vi "GUI_HTT_save.vi"() -> ()   [LabVIEW 2013]
uses:
  shared programs/GUI_Template/GUI_master/tcp_new_data_event.ctl
  shared programs/GUI_Template/GUI_master/tcp new data cluster.ctl
  GUI_TestStand/Fire button.ctl
panel:
  in  "Position.Axis 3::5 2":dbl caption="Mode Out z" min=-200.0 max=200.0
  in  "Position.Axis 1::4":dbl caption="Blade" min=-20.0 max=20.0
  out "Temperature::11":dbl min=0.0 max=500.0 format="%#_3f"
  out "Temperature::10":dbl min=0.0 max=500.0 format="%#_3f"
  out "Energy.Channel 0::7":dbl min=0.0 max=20.0 format="%#_3e"
  in  "Amplitude.Ch 5::8":dbl caption="Trigger Amplitude" min=0.0 max=12.0
  in  "Position.Axis 3::5":dbl caption="Mode In z" min=-200.0 max=200.0
  in  "Position.Axis 1::5":dbl caption="Mode Out Wedge" min=-150.0 max=150.0
  out "Position.Axis3::2":dbl caption="Rotation G1" min=-180.0 max=180.0 format="%#_13g"
  out "Position.Axis2::2":dbl caption="Rotation G2" min=-180.0 max=180.0 format="%#_13g"
  in  "Position.Axis1::2":dbl caption="Translation" min=-60000.0 max=60000.0 format="%#_13g"
  in  "PicoL":bool caption="PicoL GUI"
  in  "PicoB":bool caption="PicoB GUI"
  in  "AnalogOutput.Channel 0::9":dbl caption="Pressure Ctrl (V)" min=0.0 max=10.0
  in  "Width.Ch 5::8":dbl caption="Opening time (s)" min=0.0 max=0.025 format="%#_6e"
  in  "Jet enable":bool caption="Jet Enable"
  in  "Jet trigger":bool caption="Jet Trigger"
  in  "Position.Axis 3::3":dbl caption="Jet z" min=0.0 max=25.0
  in  "Position.Axis 2::3":dbl caption="Jet y" min=0.0 max=25.0
  in  "Position.Axis 1::3":dbl caption="Jet X" min=0.0 max=25.0
  in  "Position.Axis 3::6":dbl caption="Probe delay" min=-76.0 max=76.0
  in  "GUIdevice 11":string="HTT-Temp-Amps"
  in  "GUIdevice 8":string="HTT-BNC"
  in  "GUIdevice 6":string="HTT-ESP04"
  in  "GUIdevice 5":string="HTT-ESP03"
  in  "Fire Button":T1=TRUE
  out "error IO 2":errorcluster
  out "fire::10":string
  out "tcp data event":T2
  in  "UDP error message":string
  in  "GUIdevice 7":string="HTT-Pulsar"
  in  "GUIdevice 2":string="HTT-Aerotech"
  in  "GUIdevice 10":string="HTT-Temp-Gaia"
  in  "GUIdevice 4":string="HTT-ESP02"
  in  "GUIdevice 1":string="U_1Wire_148"
  in  "GUIdevice 3":string="HTT-ESP01"
  in  "GUIdevice 9":string="HTT-HighPressureDAQ"
  in  "Delay.Ch 5::8":dbl caption="Jet timing (s)" min=0.0 max=10.0 format="%#_6e"
  in  "stop":bool
  # "Energy"
  # "CAP"
  # "HTT CONTROL CENTER"
  # "Drive"
  # "Gas Jet"
  # "Compressor"
  # "Mode Imager"
  # "Temp Gaia"
  # "Temp Amp"
  # "Energy"
  # "Prepulse Delay"
  # "Scatter (soon)"
  # "GUI Collection"
  # "Probe"
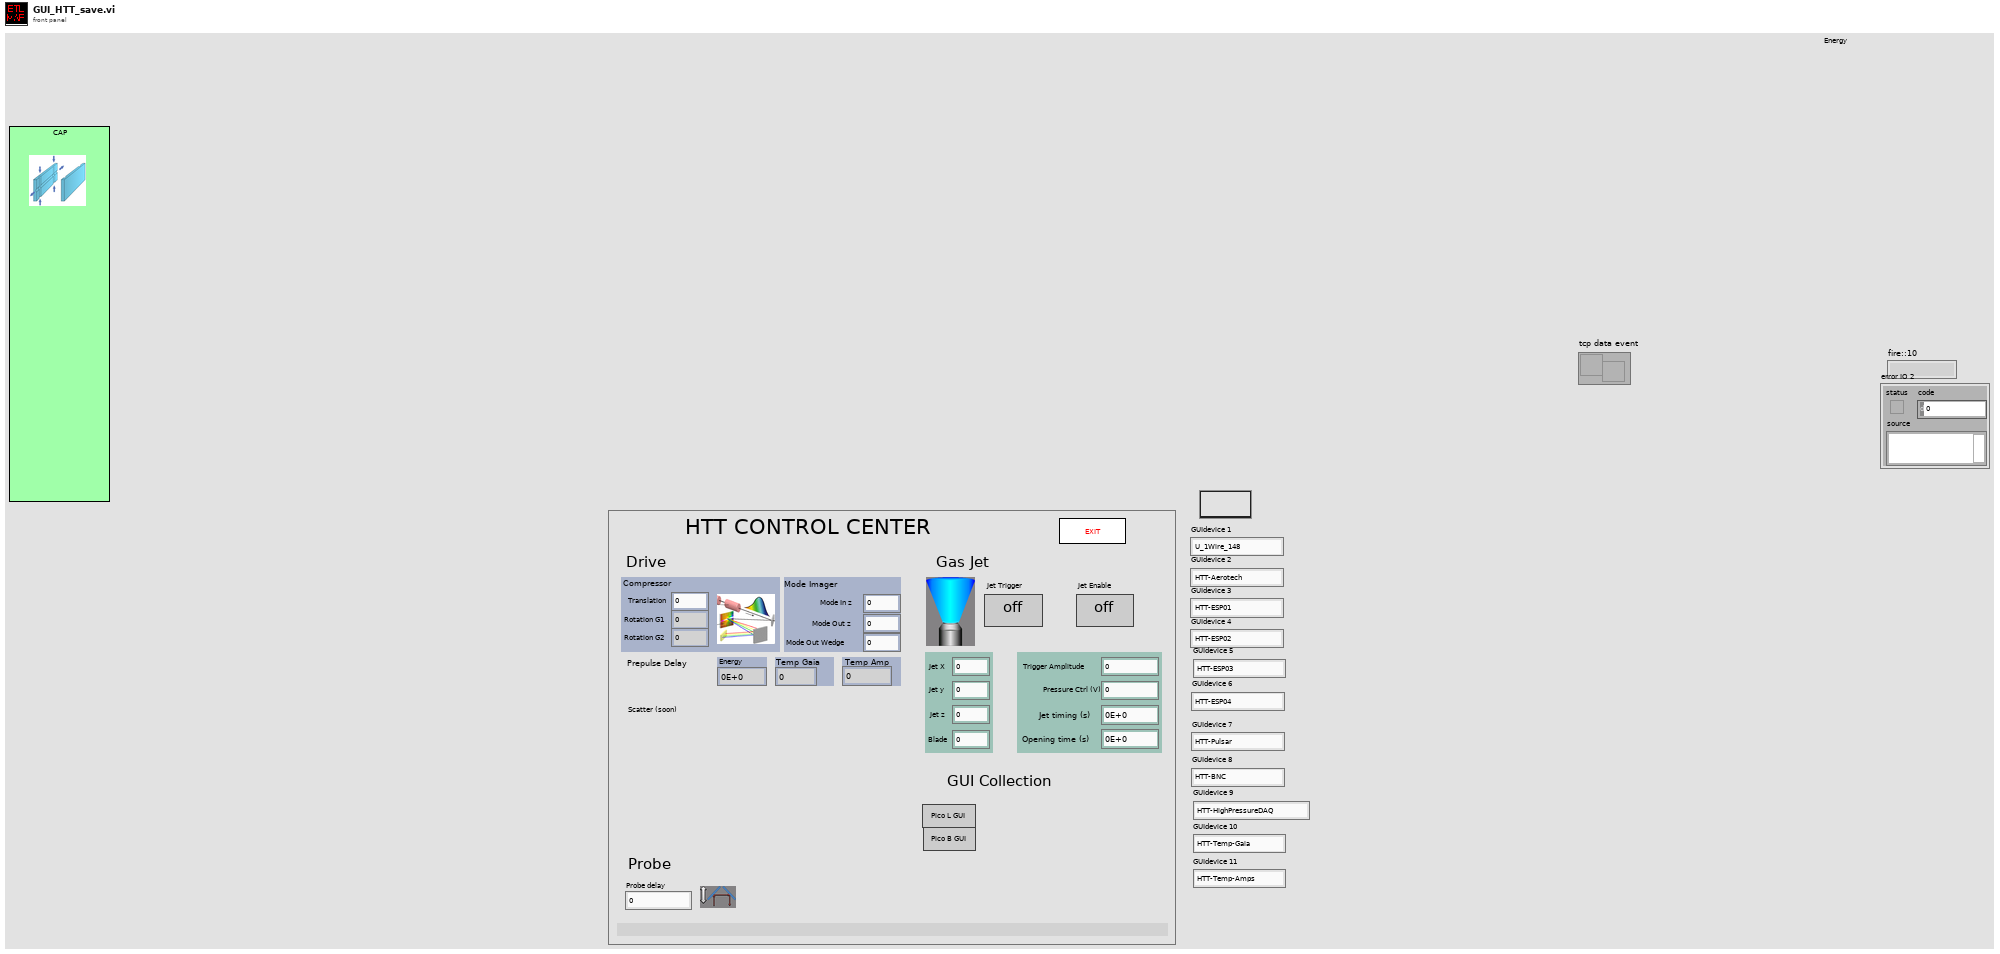
[diagram p1: front panel]
types:
  T1 = typedef "Fire button.ctl" = bool
  T2 = typedef "tcp_new_data_event.ctl" = refnum<user-event>
  T3 = typedef "tcp new data cluster.ctl" = cluster{"EventEnum":enum16{"new data", "connection status update"}, "Device name":string}
  T4 = enum32{"invalid app kind", "Development System", "Run Time System", "Student Edition", "Embedded LabVIEW", "Evaluation", "Custom"}
  T5 = enum32{"Invalid", "Standard", "Closed", "Hidden", "Minimized", "Maximized"}
  T6 = cluster{"Core":cluster{"Current VI Reference":refnum<vi>, "Close Panel on Exit?":bool}, "Heater timing offset":dbl, "Discharge timing offset":dbl, "Jet trigger":bool, "Tik1":u32, "Tik2":u32, "Fire Continues Allowed":bool, "Jet enable":bool}
  T7 = cluster{"Current VI Reference":refnum<vi>, "Close Panel on Exit?":bool}
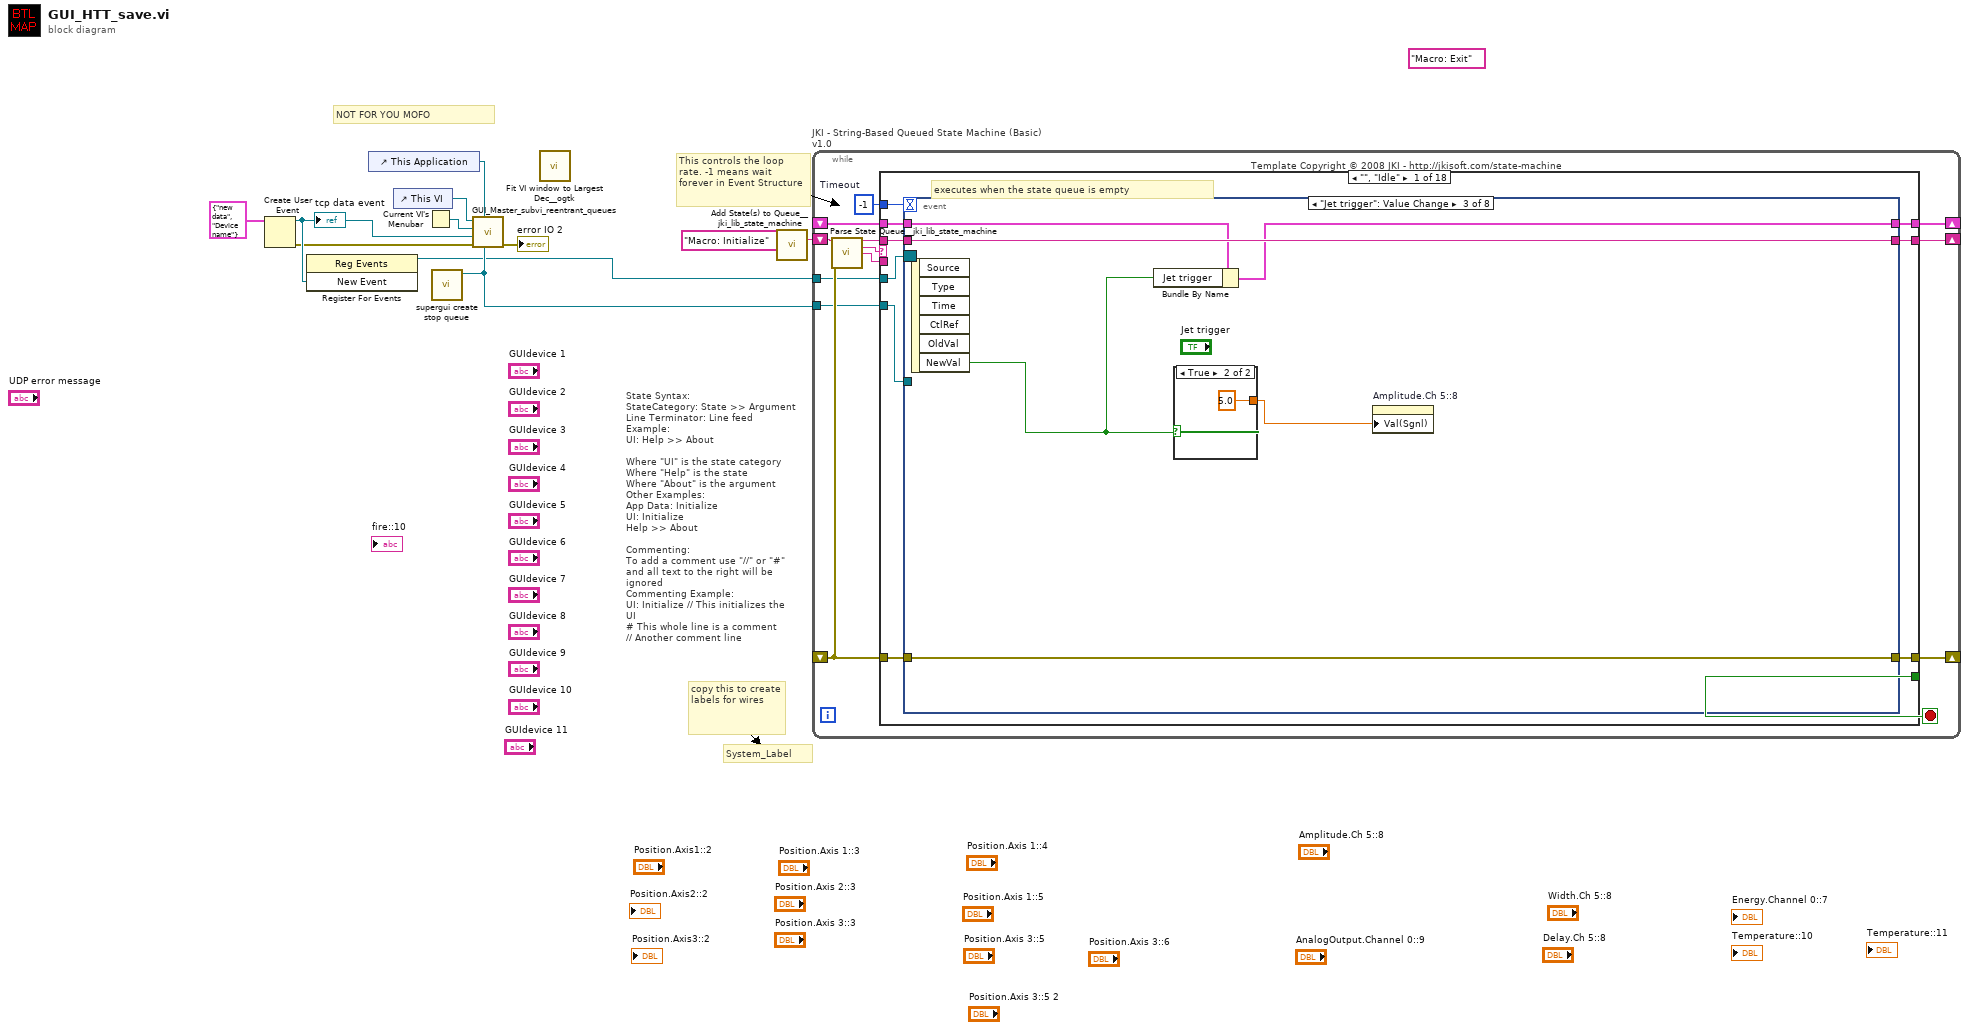
[diagram p0: block diagram]
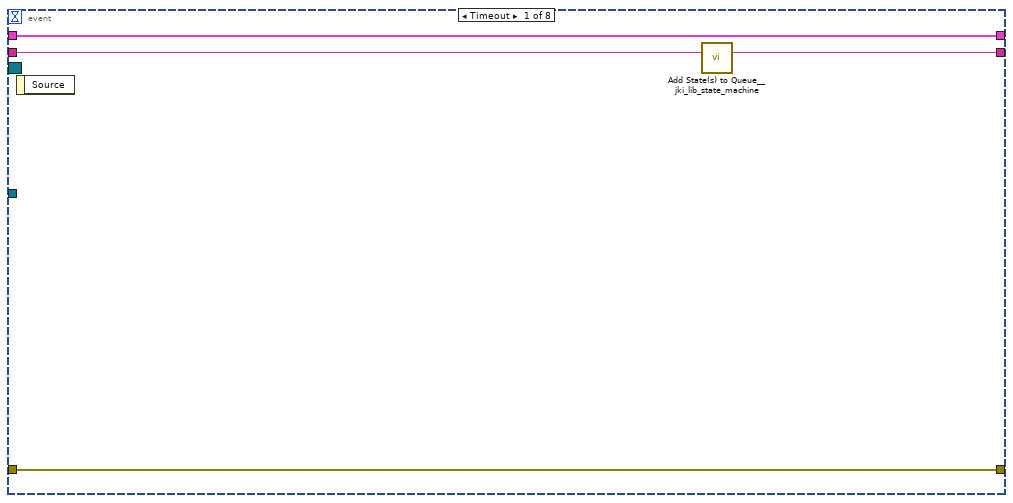
[diagram p2: hidden frame]
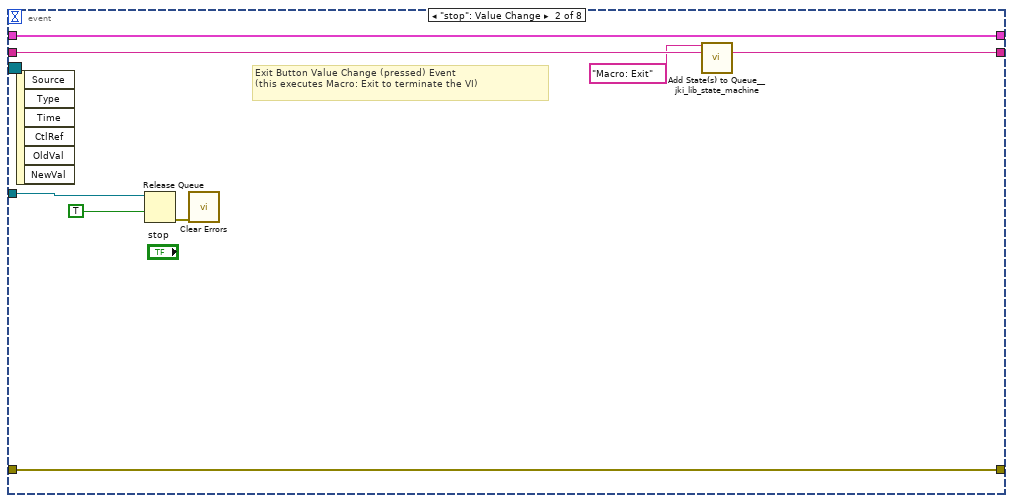
[diagram p3: hidden frame]
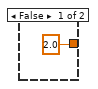
[diagram p4: hidden frame]
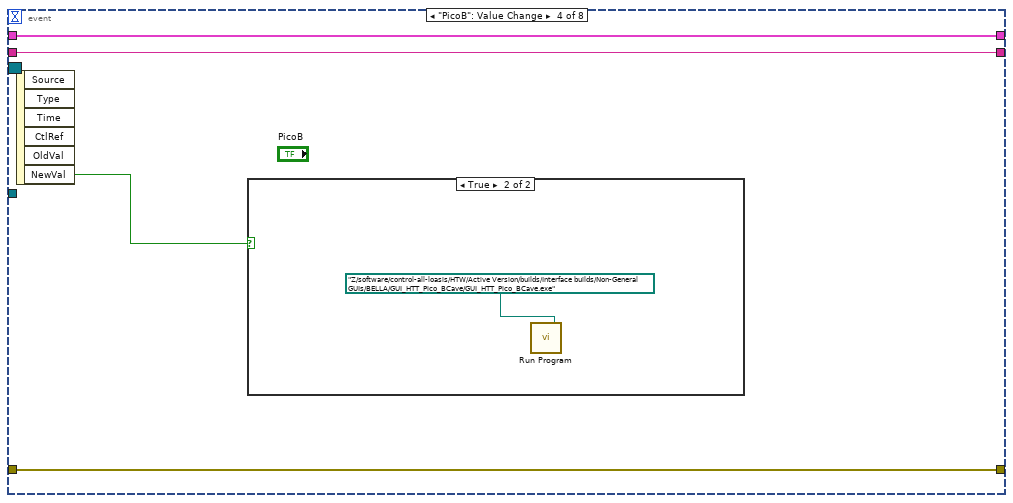
[diagram p5: hidden frame]
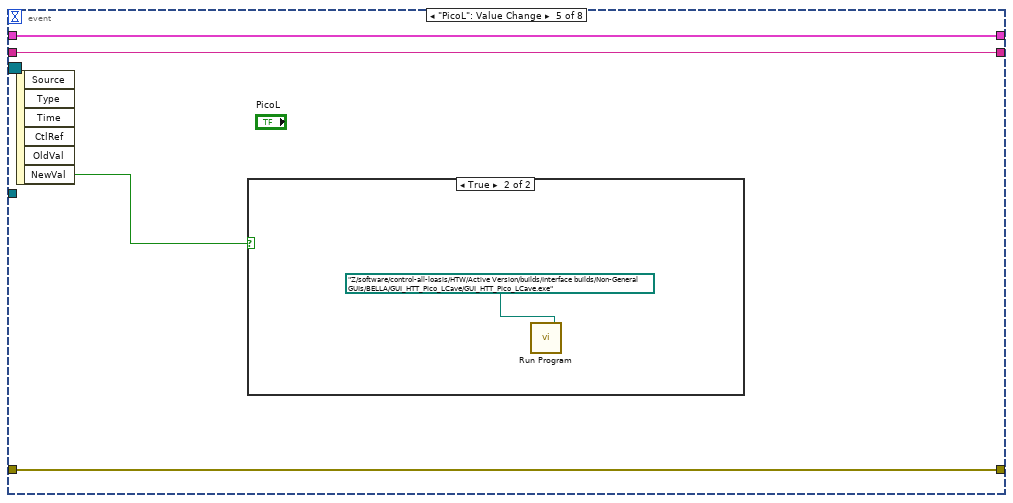
[diagram p7: hidden frame]
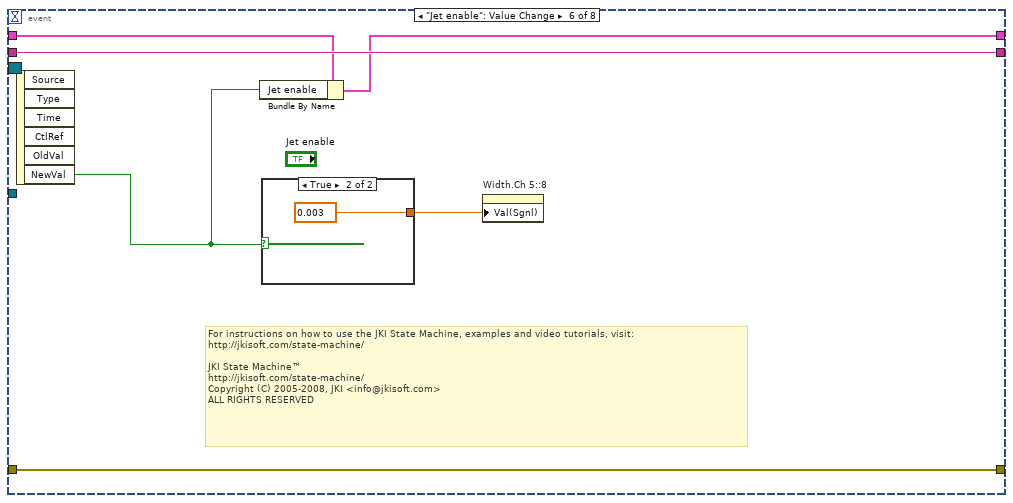
[diagram p9: hidden frame]
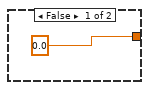
[diagram p10: hidden frame]
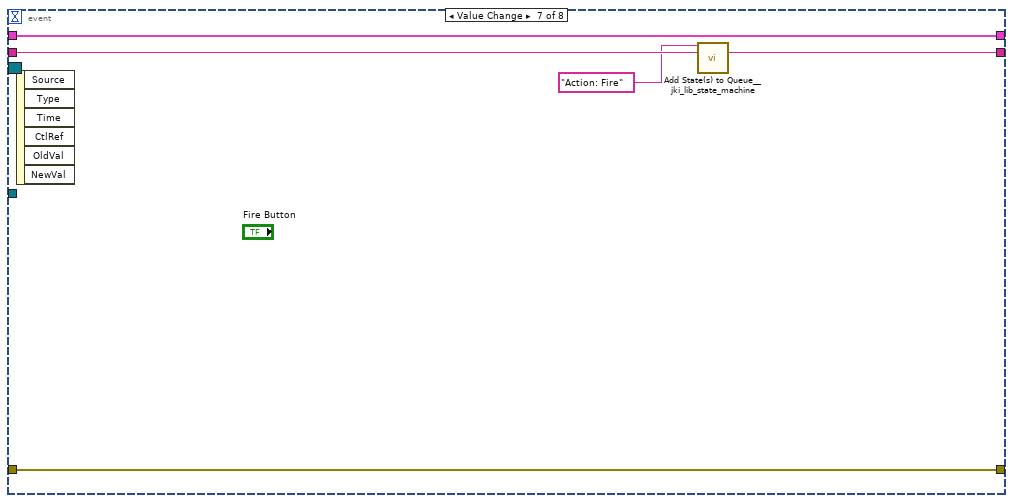
[diagram p11: hidden frame]
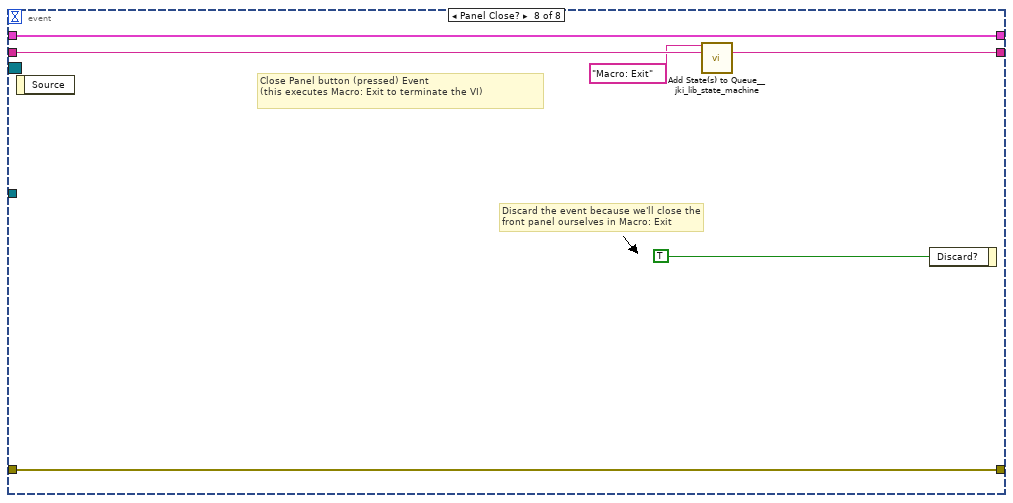
[diagram p12: hidden frame]
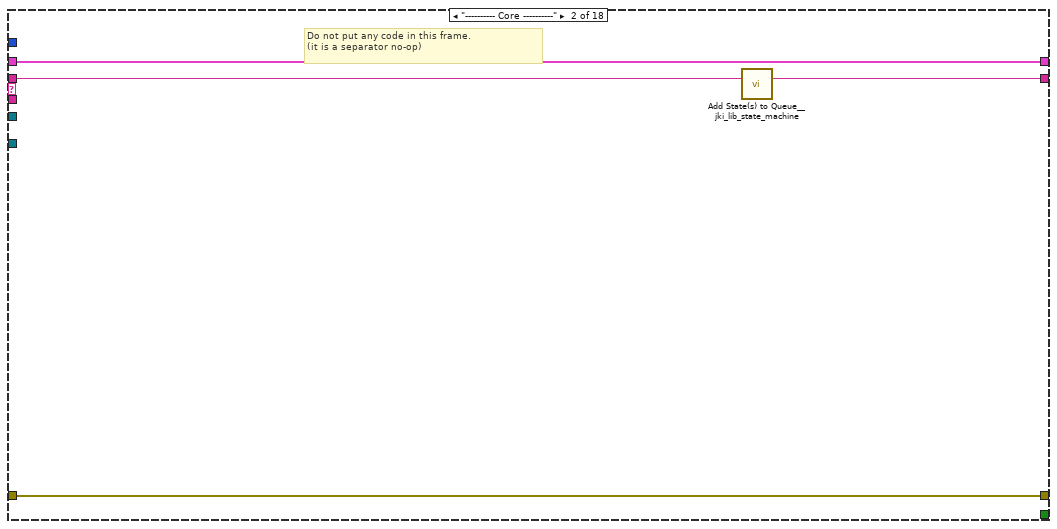
[diagram p13: hidden frame]
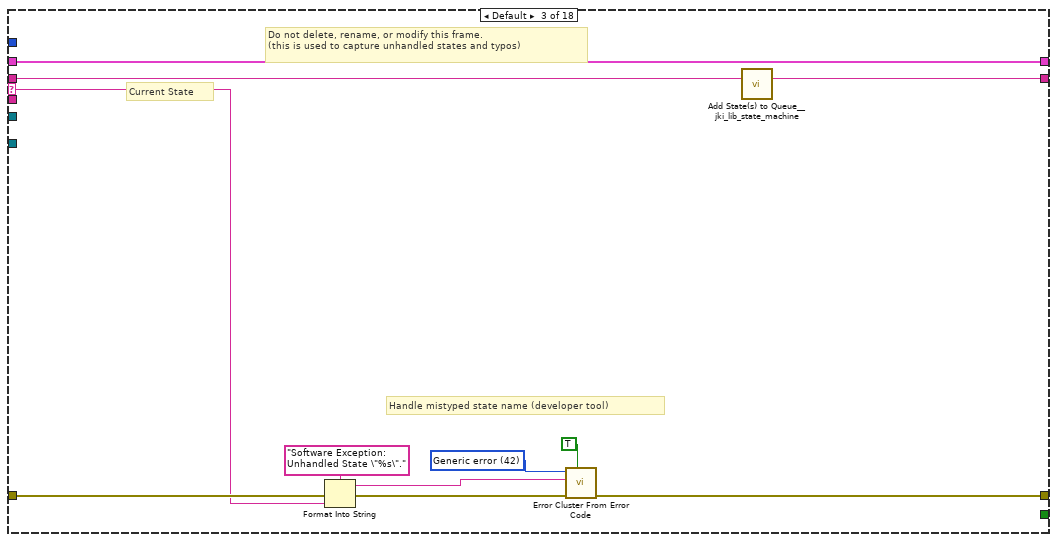
[diagram p14: hidden frame]
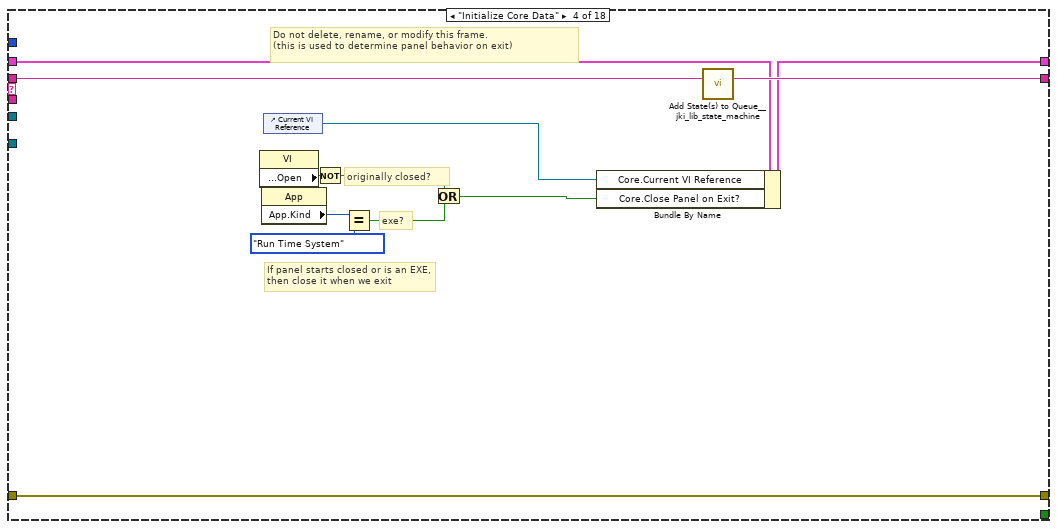
[diagram p15: hidden frame]
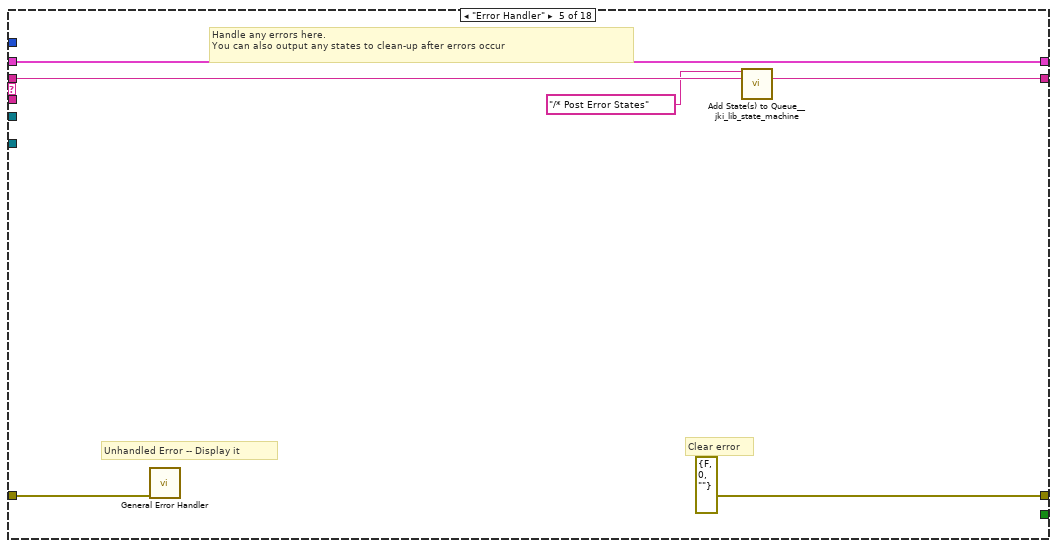
[diagram p16: hidden frame]
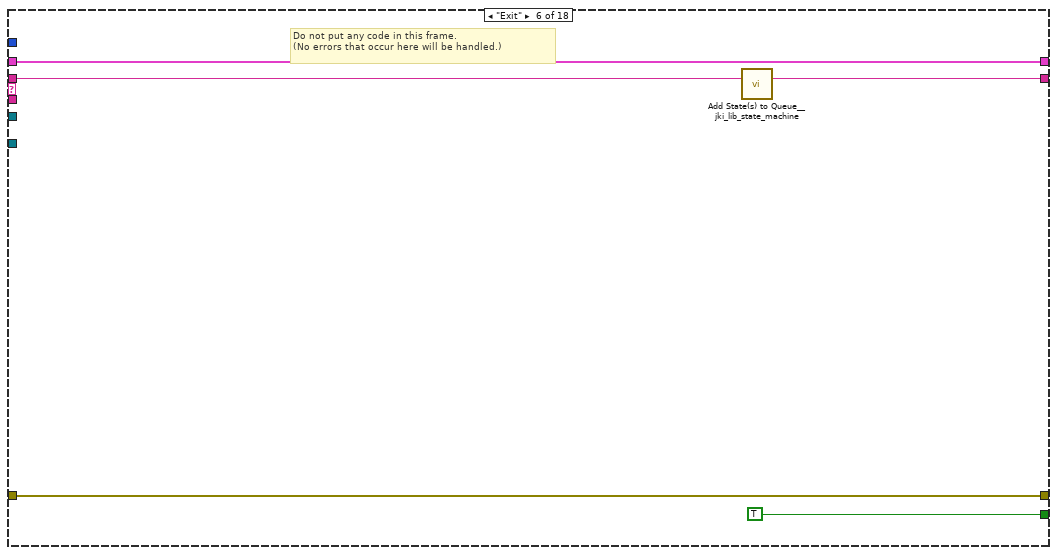
[diagram p17: hidden frame]
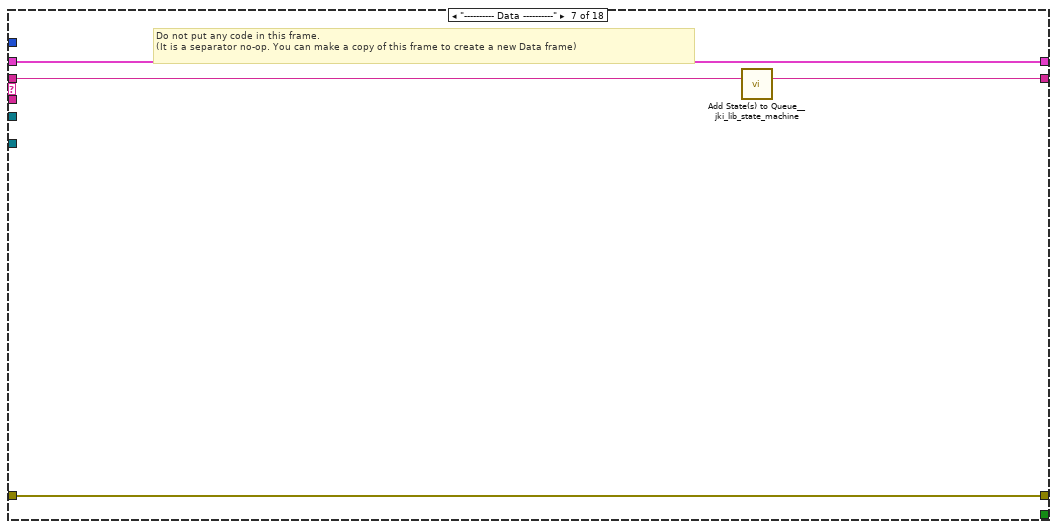
[diagram p18: hidden frame]
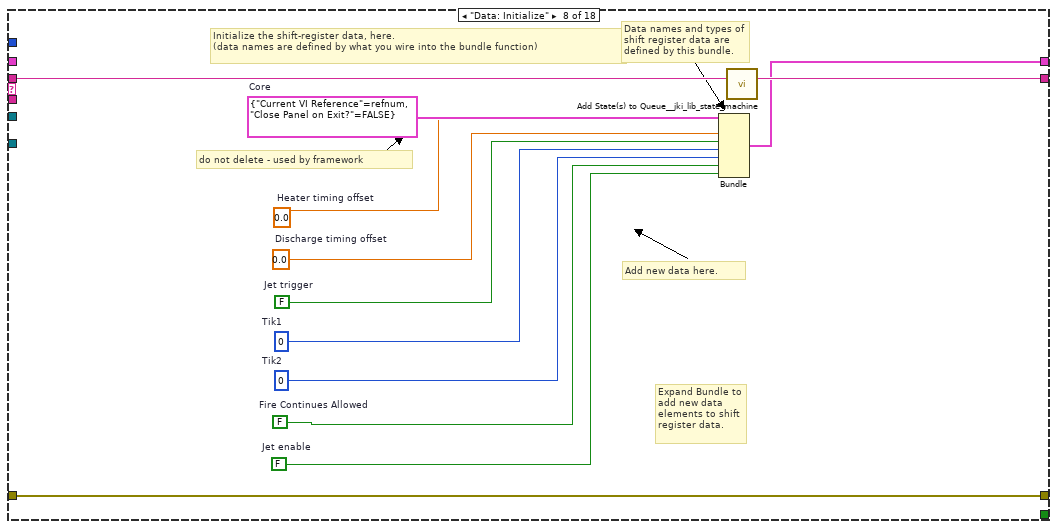
[diagram p19: hidden frame]
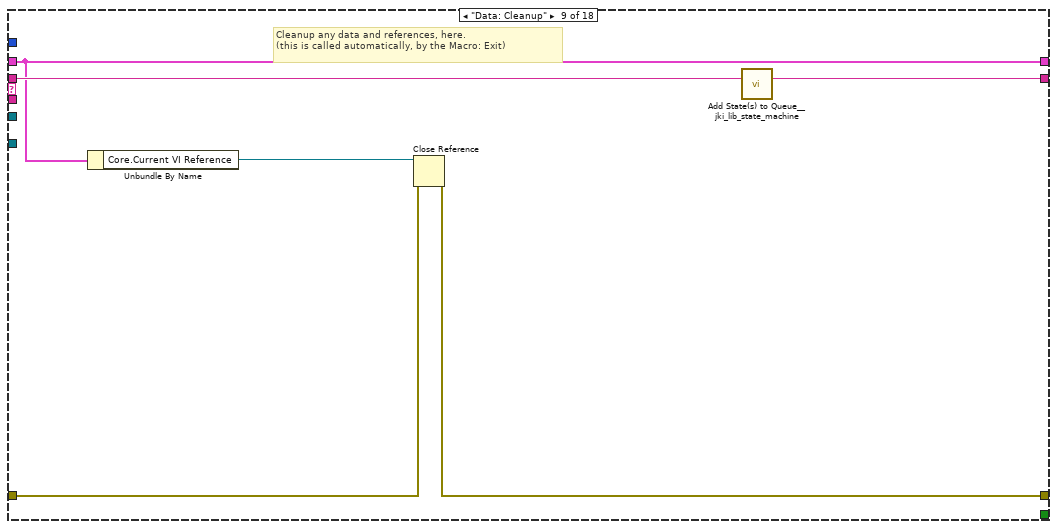
[diagram p20: hidden frame]
diagram:
  (unwired) "Macro: Exit"
  # "State Syntax:\nStateCategory: State >> Argument\nLine Terminator: Line feed\nExample:\nUI: Help >> About\n\nWhere \"UI\" is the state category\nWhere \"Help\" is the state\nWhere \"About\" is the argument\nOther Examples:\nApp Data: Initialize\nUI: Initialize\nHelp >> About\n\nCommenting:\nTo add a comment use \"//\" or \"#\" and all text to the right will be ignored\nCommenting Example:\nUI: Initialize // This initializes the UI\n# This whole line is a comment\n// Another comment line"
  # "copy this to create labels for wires"
  # "This controls the loop rate. -1 means wait forever in Event Structure"
  # "System_Label"
  # "NOT FOR YOU MOFO"
  n1 = Create User Event(user event datatype=T3 {"EventEnum"=enum."new data", "Device name"="Device name"} ("New Event")) -> (user event=w10:refnum<user-event>, error out=w9:errorcluster)  [unwired: 1 in]
  "tcp data event" <- w10
  n2 = register-events(w10) -> (reference out=w1:refnum<event-registration>)  [unwired: 2 in, 1 out]
  n3 = control-ref of="This Application"() -> (w11:refnum<vi>)
  n4 = control-ref of="This VI"() -> (w5:refnum<vi>)
  n5 = Current VI's Menubar() -> (w7:refnum<k9>)
  n6 = call "supergui create stop queue.vi"() -> ("STOP Queue out"=w2:refnum<queue>)  [unwired: 11 in]
  n7 = call "GUI_Master_subvi_reentrant_queues.vi"("STOP Queue in"=w2, "This Application"=w11, "error in (no error)"=w9, "tcp data event"=w10, "Caller menu reference"=w7, "Caller VI ref"=w5) -> ("error out"=→"error IO 2":errorcluster)  [unwired: 5 in]
  n8 = call <userlib>:"Fit VI window to Largest Dec__ogtk.vi"() -> ()  [unwired: 6 in, 2 out]
  n9 = call <vilib>:"Add State(s) to Queue__jki_lib_state_machine.vi"("State(s) in (\"\")"="Macro: Initialize") -> ("States Out"=w3:string)  [unwired: 14 in]
  n10 = while "JKI - String-Based Queued State Machine (Basic) v1.0" {
    shift-right: [w17] -> _
    shift-left: _ -> [w16]
    shift-right: [w20] -> _
    shift-left: _ -> [w14]
    shift-right: [w19] -> _
    shift-left: w3 -> [w21]
    tunnel: w1 -> [w13]
    tunnel: w2 -> [w12]
    stop <- w18 stop-if-true
    w15 = -1  # Timeout
    # "Template Copyright © 2008 JKI - http://jkisoft.com/state-machine"
    n11 = call <vilib>:"Parse State Queue__jki_lib_state_machine.vi"("State Queue"=w21, "Error In (no error)"=w14) -> ("Remaining States"=w23:string, "Current State"=w24:string, "Arguments"=w22:string)  [unwired: 11 in]
    n12 = case shown="\"\", \"Idle\"" w24 {
      selector: w24 -> [_ _ w87 _ _ _ _ _ _ _ _ _ _ _ _ _ _ _]
      tunnel: w23 -> [w33 w86 w91 w109 w115 w120 w124 w136 w142 w146 w150 w156 w167 w193 w198 w208 w212 w218]
      tunnel: w22 -> [_ _ _ _ _ _ _ _ _ _ _ w151 w161 _ _ _ _ _]
      tunnel: w16 -> [w31 w83 w89 w100 w112 w118 w121 _ w137 w143 w148 w154 w163 w190 w195 w205 w209 w216]
      tunnel: [w30 w84 w93 w106 errorcluster {"status"=FALSE, "code"=0, "source"=""} ("error out") w117 w122 w133 w138 w144 w147 w152 w164 w191 w196 w206 w210 w213] -> w20
      tunnel: w14 -> [w29 w84 w92 w106 w111 w117 w122 w133 w139 w144 w147 w153 w165 w191 w196 w206 w210 w214]
      tunnel: [w32 w85 w90 w108 w114 w119 w123 w135 w141 w145 w149 w155 w166 w192 w197 w207 w211 w217] -> w19
      tunnel: [_ _ _ _ _ TRUE _ _ _ _ _ _ _ _ _ _ _ _] -> w18
      tunnel: [w25 w83 w89 w107 w112 w118 w121 w134 w137 w143 w148 w154 w163 w190 w195 w205 w209 w216] -> w17
      tunnel: w15 -> [w28 _ _ _ _ _ _ _ _ _ _ _ _ _ _ _ _ _]
      tunnel: w13 -> [w27 _ _ _ _ _ _ _ _ _ _ _ _ _ _ _ _ _]
      tunnel: w12 -> [w26 _ _ _ _ _ _ _ _ _ _ _ _ _ _ _ _ _]
      frame "", "Idle" {
        # "executes when the state queue is empty"
        n13 = event shown="[2] \"Jet trigger\": Value Change" {
          selector: w27 -> [_ _ _ _ _ _ _ _]
          dyn-events: _ -> [_ _ _ _ _ _ _ _]
          timeout: w28 -> [_ _ _ _ _ _ _ _]
          tunnel: w33 -> [w37 w45 w51 w57 w62 w69 w73 w82]
          tunnel: [w36 w44 w51 w57 w62 w69 w74 w81] -> w32
          tunnel: w31 -> [w34 w42 w50 w54 w59 w68 w76 w79]
          tunnel: [w35 w43 w47 w55 w60 w64 w75 w80] -> w30
          tunnel: w29 -> [w35 w43 w47 w55 w60 w64 w75 w80]
          tunnel: [w34 w42 w49 w54 w59 w67 w76 w79] -> w25
          tunnel: w26 -> [_ w39 _ _ _ _ _ _]
          event Timeout {
            n14 = event-data() -> ()  [unwired: 1 in, 1 out]
            n15 = call <vilib>:"Add State(s) to Queue__jki_lib_state_machine.vi"("State(s) in (\"\")"=w37) -> ("States Out"=w36:string)  [unwired: 14 in]
          }
          event "stop": Value Change {
            # "Exit Button Value Change (pressed) Event\n(this executes Macro: Exit to terminate the VI)"
            n16 = event-data() -> ()  [unwired: 1 in, 6 out]
            n17 = Release Queue(queue=w39, force destroy? (F)=TRUE) -> (error out=w40:errorcluster)  [unwired: 1 in, 2 out]
            n18 = call <vilib>:"Clear Errors.vi"("error in (no error)"=w40) -> ()  [unwired: 6 in, 1 out]
            n19 = call <vilib>:"Add State(s) to Queue__jki_lib_state_machine.vi"("State(s) in Front (\"\")"="Macro: Exit", "State(s) in (\"\")"=w45) -> ("States Out"=w44:string)  [unwired: 13 in]
          }
          event "Jet trigger": Value Change {
            n20 = event-data() -> ("NewVal"=w48:bool)  [unwired: 1 in, 5 out]
            n21 = Bundle By Name(cluster=w50, "Jet trigger"=w48) -> (w49:T6)
            n22 = case shown="True" w48 {
              tunnel: [2.0 ("Amplitude.Ch CD::10") 5.0 ("Amplitude.Ch CD::10")] -> w46
              frame False {
              }
              frame True {
              }
            }
            n23 = property on="Amplitude.Ch 5::8" class="DigNum (strict)"("Val(Sgnl)"=w46) -> ()  [unwired: 2 in, 2 out]
          }
          event "PicoB": Value Change {
            n24 = event-data() -> ("NewVal"=w56:bool)  [unwired: 1 in, 5 out]
            n25 = case shown="True" w56 {
              frame False {
              }
              frame True {
                n26 = call "Run Program.vi"("Program Path"=path "Z:/software/control-all-loasis/HTW/Active Version/builds/Interface builds/Non-General GUIs/BELLA/GUI_HTT_Pico_BCave/GUI_HTT_Pico_BCave.exe") -> ()  [unwired: 1 in]
              }
            }
          }
          event "PicoL": Value Change {
            n27 = event-data() -> ("NewVal"=w61:bool)  [unwired: 1 in, 5 out]
            n28 = case shown="True" w61 {
              frame False {
              }
              frame True {
                n29 = call "Run Program.vi"("Program Path"=path "Z:/software/control-all-loasis/HTW/Active Version/builds/Interface builds/Non-General GUIs/BELLA/GUI_HTT_Pico_LCave/GUI_HTT_Pico_LCave.exe") -> ()  [unwired: 1 in]
              }
            }
          }
          event "Jet enable": Value Change {
            # "For instructions on how to use the JKI State Machine, examples and video tutorials, visit:\nhttp://jkisoft.com/state-machine/\n\nJKI State Machine™\nhttp://jkisoft.com/state-machine/\nCopyright (C) 2005-2008, JKI <info@jkisoft.com>\nALL RIGHTS RESERVED"
            n30 = event-data() -> ("NewVal"=w66:bool)  [unwired: 1 in, 5 out]
            n31 = Bundle By Name(cluster=w68, "Jet enable"=w66) -> (w67:T6)
            n32 = case shown="True" w66 {
              tunnel: [0.0 ("opening Time") 0.003 ("opening Time")] -> w65
              frame False {
              }
              frame True {
              }
            }
            n33 = property on="Width.Ch 5::8" class="DigNum (strict)"("Val(Sgnl)"=w65) -> ()  [unwired: 2 in, 2 out]
          }
          event Value Change {
            n34 = event-data() -> ()  [unwired: 1 in, 6 out]
            n35 = call <vilib>:"Add State(s) to Queue__jki_lib_state_machine.vi"("State(s) in Front (\"\")"="Action: Fire" ("State(s) in Front (\"\")"), "State(s) in (\"\")"=w73) -> ("States Out"=w74:string)  [unwired: 13 in]
          }
          event Panel Close? {
            # "Discard the event because we'll close the front panel ourselves in Macro: Exit"
            # "Close Panel button (pressed) Event\n(this executes Macro: Exit to terminate the VI)"
            n36 = event-data() -> ()  [unwired: 1 in, 1 out]
            n37 = call <vilib>:"Add State(s) to Queue__jki_lib_state_machine.vi"("State(s) in Front (\"\")"="Macro: Exit", "State(s) in (\"\")"=w82) -> ("States Out"=w81:string)  [unwired: 13 in]
            n38 = event-data("Discard?"=TRUE) -> ()  [unwired: 1 in, 1 out]
          }
        }
      }
      frame "---------- Core ----------" {
        # "Do not put any code in this frame.\n(it is a separator no-op)"
        n39 = call <vilib>:"Add State(s) to Queue__jki_lib_state_machine.vi"("State(s) in (\"\")"=w86) -> ("States Out"=w85:string)  [unwired: 14 in]
      }
      frame Default {
        w96 = 42 items=["No error", "Argument error", "Memory is full", "Out of zone", "End of file", "File already open", "Generic file I/O error", "File not found", "File permission error", "Disk is full", "Duplicate path", "Too many files open", "System feature not enabled", "Resource file not found", "Cannot add resource", "Resource not found", "Image not found", "Image memory error", "Pen does not exist", "Config type invalid", "Config token not found", "Config parse error", "Config memory error", "Bad external code format", "Bad external code offset", "External code not present", "Null window", "Destroy window error", "Null menu", "Print aborted", "Bad print record", "Print driver error", "Windows error during printing", "Memory error during printing", "Print dialog error", "Generic print error", "Invalid device refnum", "Device not found", "Device parameter error", "Device unit error", "Cannot open device", "Device call aborted", "Generic error", "Cancelled by user", "Object ID too low", "Object ID too high", "Object not in heap", "Unknown heap", "Unknown object (invalid DefProc)", "Unknown object (DefProc not in table)", "Message out of range", "Invalid (null) method", "Unknown message", "Manager call not supported", "Bad address", "Network operation in progress", "Network operation timed out", "Connection is busy", "Network attribute not supported", "Network error", "Address in use", "System out of memory", "Connection aborted", "Connection refused", "Not connected", "Already connected", "Connection closed", "Initialization error (interapplication manager)", "Bad occurrence", "Wait on unbound occurrence handler", "Occurrence queue overflow", "Datalog type conflict", "Unused", "Unrecognized type (interapplication manager)", "Memory corrupt", "Failed to make temporary DLL", "Old CIN version", "Drag socket not found", "Failed to load drop-object", "Failed to register OLE object", "Failed to release OLE object", "Format specifier type mismatch", "Unknown format specifier", "Too few format specifiers", "Too many format specifiers", "Scan failed", "Newer CIN version", "Error converting to variant", "Runtime menu error", "Password tampered", "Variant attribute not found", "Incompatible variant data type", "Event data is not available", "Event Store is not present", "Occurrence is not found", "Event Queue is not created", "Event info is not available", "Refnum passed is NULL", "Error retrieving Class GUID", "Error retrieving CoClass GUID", "Error retrieving TypeLib GUID.", "Bad built application magic bytes.", "Specific driver is different from the specific driver associated with the Logical Name.", "There is no session opened to the class driver.", "Max Error", "MAX - Error with config objects", "MAX - Error loading configuration", "MAX - Group not supported"]
        # "Current State"
        # "Do not delete, rename, or modify this frame.\n(this is used to capture unhandled states and typos)"
        # "Handle mistyped state name (developer tool)"
        n40 = Format Into String(format string="Software Exception: Unhandled State \"%s\"." ("message"), error in=w92, w87) -> (resulting string=w95:string, error out=w94:errorcluster)  [unwired: 1 in]
        n41 = call <vilib>:"Error Cluster From Error Code.vi"("show call chain? (False)"=TRUE, "error in (no error)"=w94, "error message (\"\")"=w95, "error code (0)"=w96) -> ("error out"=w93:errorcluster)  [unwired: 5 in]
        n42 = call <vilib>:"Add State(s) to Queue__jki_lib_state_machine.vi"("State(s) in (\"\")"=w91) -> ("States Out"=w90:string)  [unwired: 14 in]
      }
      frame "Initialize Core Data" {
        # "Do not delete, rename, or modify this frame.\n(this is used to determine panel behavior on exit)"
        # "originally closed?"
        # "exe?"
        # "If panel starts closed or is an EXE, then close it when we exit"
        n43 = property class="VI"() -> ("Front Panel.Open"=w105:bool)  [unwired: 2 in, 2 out]
        n44 = property class="App"() -> ("App.Kind"=w104:T4)  [unwired: 2 in, 2 out]
        n45 = control-ref of="Current VI Reference"() -> (w98:refnum<vi>)
        n46 = Not(x=w105) -> (.not. x?=w102:bool)
        n47 = Equal?(x=w104, y=T4."Run Time System" ("Application:Kind")) -> (x = y?=w101:bool)
        n48 = Or(x=w102, y=w101) -> (x .or. y?=w99:bool)
        n49 = Bundle By Name(cluster=w100, "Core.Current VI Reference"=w98, "Core.Close Panel on Exit?"=w99) -> (w107:T6)
        n50 = call <vilib>:"Add State(s) to Queue__jki_lib_state_machine.vi"("State(s) in (\"\")"=w109) -> ("States Out"=w108:string)  [unwired: 14 in]
      }
      frame "Error Handler" {
        # "Unhandled Error -- Display it"
        # "Handle any errors here.\nYou can also output any states to clean-up after errors occur"
        # "Clear error"
        n51 = call <vilib>:"General Error Handler.vi"("error in (no error)"=w111) -> ()  [unwired: 10 in, 5 out]
        n52 = call <vilib>:"Add State(s) to Queue__jki_lib_state_machine.vi"("State(s) in Front (\"\")"="/* Post Error States", "State(s) in (\"\")"=w115) -> ("States Out"=w114:string)  [unwired: 13 in]
      }
      frame "Exit" {
        # "Do not put any code in this frame.\n(No errors that occur here will be handled.)"
        n53 = call <vilib>:"Add State(s) to Queue__jki_lib_state_machine.vi"("State(s) in (\"\")"=w120) -> ("States Out"=w119:string)  [unwired: 14 in]
      }
      frame "---------- Data ----------" {
        # "Do not put any code in this frame.\n(It is a separator no-op. You can make a copy of this frame to create a new Data frame)"
        n54 = call <vilib>:"Add State(s) to Queue__jki_lib_state_machine.vi"("State(s) in (\"\")"=w124) -> ("States Out"=w123:string)  [unwired: 14 in]
      }
      frame "Data: Initialize" {
        w125 = FALSE  # Jet enable
        w126 = FALSE  # Fire Continues Allowed
        w128 = u32 0  # Tik1
        w127 = u32 0  # Tik2
        w129 = FALSE  # Jet trigger
        w130 = 0.0  # Discharge timing offset
        w131 = 0.0  # Heater timing offset
        w132 = T7 {"Current VI Reference"=refnum, "Close Panel on Exit?"=FALSE}  # Core
        # "do not delete - used by framework"
        # "Expand Bundle to add new data elements to shift register data."
        # "Add new data here."
        # "Data names and types of shift register data are defined by this bundle."
        # "Initialize the shift-register data, here.\n(data names are defined by what you wire into the bundle function)"
        n55 = Bundle("Core"=w132, "Heater timing offset"=w131, "Discharge timing offset"=w130, "Jet trigger"=w129, "Tik1"=w128, "Tik2"=w127, "Fire Continues Allowed"=w126, "Jet enable"=w125) -> (w134:T6)  [unwired: 1 in]
        n56 = call <vilib>:"Add State(s) to Queue__jki_lib_state_machine.vi"("State(s) in (\"\")"=w136) -> ("States Out"=w135:string)  [unwired: 14 in]
      }
      frame "Data: Cleanup" {
        # "Cleanup any data and references, here.\n(this is called automatically, by the Macro: Exit)"
        n57 = Unbundle By Name(w137) -> ("Core.Current VI Reference"=w140:refnum<vi>)
        n58 = Close Reference(reference=w140, error in (no error)=w139) -> (error out=w138:errorcluster)
        n59 = call <vilib>:"Add State(s) to Queue__jki_lib_state_machine.vi"("State(s) in (\"\")"=w142) -> ("States Out"=w141:string)  [unwired: 14 in]
      }
      frame "---------- UI ----------" {
        # "Do not put any code in this frame.\n(It is a separator no-op. You can make a copy of this frame to create a new UI frame)"
        n60 = call <vilib>:"Add State(s) to Queue__jki_lib_state_machine.vi"("State(s) in (\"\")"=w146) -> ("States Out"=w145:string)  [unwired: 14 in]
      }
      frame "UI: Initialize" {
        # "Initialize the User Interface, here.\n(this is called automatically, by the Macro: Init)"
        n61 = call <vilib>:"Add State(s) to Queue__jki_lib_state_machine.vi"("State(s) in (\"\")"=w150) -> ("States Out"=w149:string)  [unwired: 14 in]
      }
      frame "UI: Cursor Set" {
        # "Argument"
        # "Set and Unset Cursor Busy.\n(Usage: \"UI: Cursor Set >> Busy|Idle\")"
        n62 = case shown="\"Idle\", Default" w151 {
          tunnel: w153 -> [w158 w160]
          tunnel: [w157 w159] -> w152
          frame "Idle", Default {
            n63 = call <vilib>:"Unset Busy.vi"("error in (no error)"=w158) -> ("error out"=w157:errorcluster)  [unwired: 10 in]
          }
          frame "Busy" {
            n64 = call <vilib>:"Set Busy.vi"("error in (no error)"=w160) -> ("error out"=w159:errorcluster)  [unwired: 9 in, 1 out]
          }
        }
        n65 = call <vilib>:"Add State(s) to Queue__jki_lib_state_machine.vi"("State(s) in (\"\")"=w156) -> ("States Out"=w155:string)  [unwired: 14 in]
      }
      frame "UI: Front Panel State" {
        # "Argument"
        # "Set Front Panel Open or Closed\n(Usage: \"UI: Front Panel State >> Open|Close\")"
        n66 = Unbundle By Name(w163) -> ("Core.Current VI Reference"=w162:refnum<vi>)
        n67 = case shown="\"Close\"" w161 {
          tunnel: w165 -> [w171 w184]
          tunnel: [w173 w185] -> w164
          tunnel: w162 -> [w172 w182]
          frame "Open", Default {
            n68 = property class="VI"(reference=w172, error in=w171) -> (reference out=w169:refnum<vi>, error out=w170:errorcluster, "Front Panel.Open"=w168:bool)
            n69 = case shown="False" w168 {
              tunnel: [w176 w179] -> w173
              tunnel: w170 -> [w175 w179]
              tunnel: w169 -> [w174 _]
              frame False {
                n70 = invoke class="VI" method="FP.Open"(reference=w174, error in=w175, "Activate"=TRUE, "State"=T5."Standard") -> (error out=w176:errorcluster)  [unwired: 1 in, 4 out]
              }
              frame True {
              }
            }
          }
          frame "Close" {
            n71 = property class="VI"(reference=w182, error in=w184) -> (reference out=w181:refnum<vi>, error out=w183:errorcluster, "Front Panel.Open"=w180:bool)
            n72 = case shown="True" w180 {
              tunnel: [w186 w189] -> w185
              tunnel: w183 -> [w186 w188]
              tunnel: w181 -> [_ w187]
              frame False {
              }
              frame True {
                n73 = invoke class="VI" method="FP.Close"(reference=w187, error in=w188) -> (error out=w189:errorcluster)  [unwired: 1 in, 2 out]
              }
            }
          }
        }
        n74 = call <vilib>:"Add State(s) to Queue__jki_lib_state_machine.vi"("State(s) in (\"\")"=w167) -> ("States Out"=w166:string)  [unwired: 14 in]
      }
      frame "---------- Macro ----------" {
        # "Do not put any code in this frame.\n(It is a separator no-op. You can make a copy of this frame to create a new Macro frame)"
        n75 = call <vilib>:"Add State(s) to Queue__jki_lib_state_machine.vi"("State(s) in (\"\")"=w193) -> ("States Out"=w192:string)  [unwired: 14 in]
      }
      frame "Macro: Initialize" {
        w194 = "Data: Initialize\nInitialize Core Data\nUI: Initialize\nUI: Front Panel State >> Open"  # Data: Initialize Initialize Core Data UI: Initialize UI: Front Panel State >> Open
        # "Initialization Macro\n(This is called once, when the VI starts)"
        n76 = call <vilib>:"Add State(s) to Queue__jki_lib_state_machine.vi"("State(s) in Front (\"\")"=w194, "State(s) in (\"\")"=w198) -> ("States Out"=w197:string)  [unwired: 13 in]
      }
      frame "Macro: Exit" {
        # "Exit Macro\n(This is called once, when the VI exits)"
        n77 = Unbundle By Name(w205) -> ("Core.Close Panel on Exit?"=w204:bool)
        n78 = Select(t="UI: Front Panel State >> Close", s=w204, f="") -> (s? t:f=w201:string)
        n79 = call <vilib>:"Add State(s) to Queue__jki_lib_state_machine.vi"("State(s) in (\"\")"=w201, "State(s) at Back (\"\")"="Data: Cleanup\nExit") -> ("States Out"=w199:string)  [unwired: 13 in]
        n80 = call <vilib>:"Add State(s) to Queue__jki_lib_state_machine.vi"("State(s) in Front (\"\")"=w199, "State(s) in (\"\")"=w208) -> ("States Out"=w207:string)  [unwired: 13 in]
      }
      frame "---------- New Category ----------" {
        # "Template Separator\n(You can make a copy of, or modify, this frame)"
        n81 = call <vilib>:"Add State(s) to Queue__jki_lib_state_machine.vi"("State(s) in (\"\")"=w212) -> ("States Out"=w211:string)  [unwired: 14 in]
      }
      frame "Action: Fire" {
        # "Your code here.\n(You can make a copy of, or modify, this frame)"
        n82 = property on="fire::10" class="Str"(error in=w214, "Val(Sgnl)"="fire>>force" ("Value (Signaling)")) -> (error out=w213:errorcluster)  [unwired: 1 in, 1 out]
        n83 = call <vilib>:"Add State(s) to Queue__jki_lib_state_machine.vi"("State(s) in (\"\")"=w218) -> ("States Out"=w217:string)  [unwired: 14 in]
      }
    }
  }
